vi "_rsscope Format Word I64.vi"(8 "error in (no error)":errorcluster, 9 "Word (1)":i64=1, 10 "Input String":string, 11 "VISA resource name":refnum<visa-resource-name>) -> (0 "error out":errorcluster, 2 "Output String":string, 3 "VISA resource name out":refnum<visa-resource-name>)   [LabVIEW 2014]
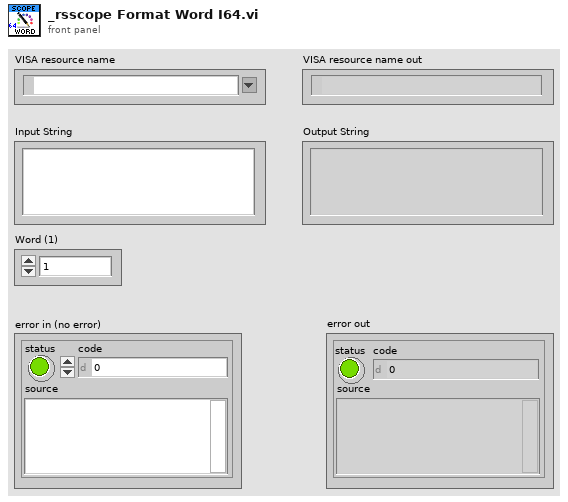
[diagram p1: front panel]
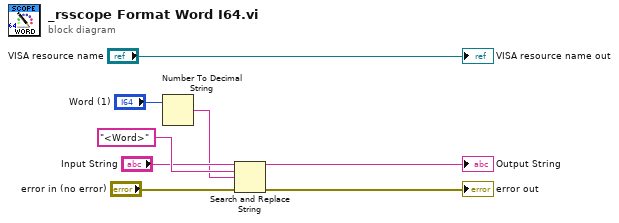
[diagram p0: block diagram]
diagram:
  n1 = Number To Decimal String(number="Word (1)") -> (decimal integer string=w5:string)  [unwired: 1 in]
  n2 = Search and Replace String(input string="Input String", search string="<Word>" ("substring (\"\")"), replace string=w5, error in="error in (no error)") -> (result string=→"Output String":string, error out=→"error out":errorcluster)  [unwired: 4 in, 2 out]
  "VISA resource name out" <- "VISA resource name"
